vi "GUI Interlock Tester.vi"(8 "Power State":bool, 9 "Self Test Button":refnum<vi>, 10 "Power Off Button":refnum<vi>, 11 "Power On Button":refnum<vi>) -> ()   [LabVIEW 2018, in "Device Under Test_Cloneable_DQMH.lvlib"]
uses:
  Device Under Test_Cloneable_DQMH.lvlib
  GUI Control References--cluster.ctl
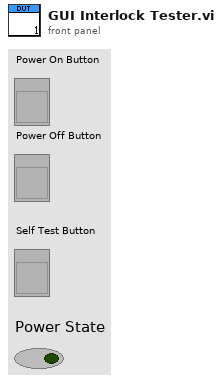
[diagram p1: front panel]
types:
  T1 = typedef "Device Under Test_Cloneable_DQMH.lvlib/GUI Control References--cluster.ctl" = cluster{"Power On Button":refnum<vi>, "Power Off Button":refnum<vi>, "Self Test Button":refnum<vi>, "Power State LED":refnum<vi>, "Self Test Result LED":refnum<vi>}
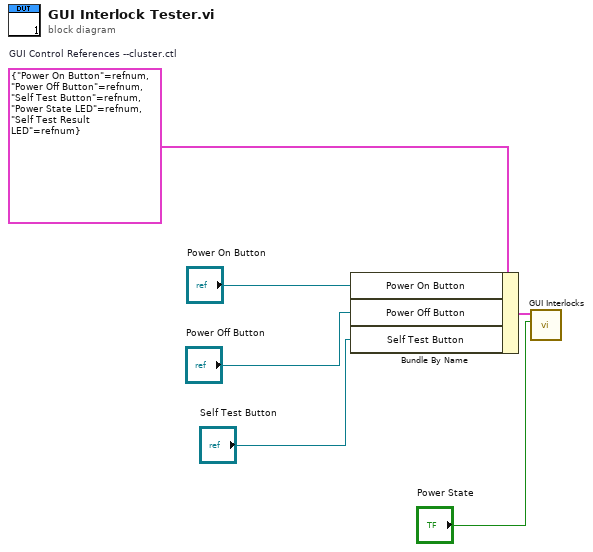
[diagram p0: block diagram]
diagram:
  w4 = T1 {"Power On Button"=refnum, "Power Off Button"=refnum, "Self Test Button"=refnum, "Power State LED"=refnum, "Self Test Result LED"=refnum}  # GUI Control References --cluster.ctl
  n1 = Bundle By Name(cluster=w4, "Power On Button"="Power On Button", "Power Off Button"="Power Off Button", "Self Test Button"="Self Test Button") -> (w5:T1)
  n2 = call "GUI Interlocks.vi"("Power State"="Power State", "References"=w5) -> ()  [unwired: 10 in]
